vi "Perform Action on Target.vi"(8 "error in":errorcluster, 9 "Input":variant, 10 "Task-Point Ident":string, 11 "Series Actor in":refnum<class "Series Actor.lvclass">) -> (0 "error out":errorcluster, 1 "Output":variant, 3 "Series Actor out":refnum<class "Series Actor.lvclass">)   [LabVIEW 2023, in "Series Actor.lvlib" / "Series Actor.lvclass"]
uses:
  Series Actor.lvclass
  <vilib>/ActorFramework/Actor/Actor.lvclass/Actor.ctl
  Study/Study Actor/IStudy Actor Messages/Perform Action on Target Msg/Perform Action on Target Msg.lvclass/Perform Action on Target Msg.ctl
  <vilib>/ActorFramework/Reply Msg/Reply Msg.lvclass/Reply Msg.ctl
  <vilib>/ActorFramework/Message Enqueuer/Message Enqueuer.lvclass/Message Enqueuer.ctl
  <vilib>/ActorFramework/Reply Msg/Send Message And Wait For Response.vi
  <vilib>/ActorFramework/Message Enqueuer/Enqueue.vi
  Study/Study Actor/IStudy Actor Messages/Perform Action on Target Msg/Perform Action on Target Msg.lvclass
  <vilib>/ActorFramework/Reply Msg/Reply Msg.lvclass
  <vilib>/Utility/LVClass/Get LV Class Name.vi
  <resource>/AFDebug/Generate Trace for Message.vi
  <vilib>/ActorFramework/Message Priority Queue/Priority Enqueue.vi
  <vilib>/ActorFramework/Actor/Actor.lvclass
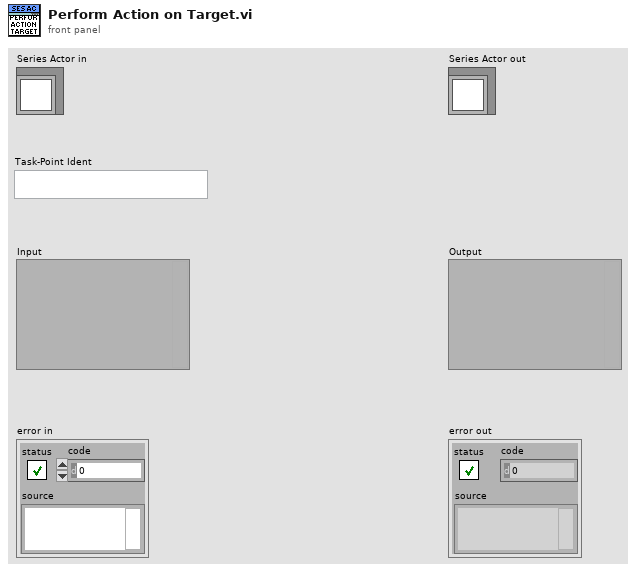
[diagram p1: front panel]
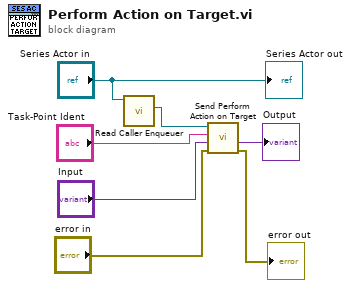
[diagram p0: block diagram]
diagram:
  n1 = call <vilib>:"Read Caller Enqueuer.vi"("Actor"="Series Actor in") -> ("Caller Enqueuer"=w4:refnum<class "Message Enqueuer.lvclass">)  [unwired: 10 in]
  n2 = call "Send Perform Action on Target.vi"("error in"="error in", "Input"="Input", "Task-Point Ident"="Task-Point Ident", "Message Enqueuer"=w4) -> ("error out"=→"error out":errorcluster, "Output"=→"Output":variant)  [unwired: 5 in, 1 out]
  "Series Actor out" <- "Series Actor in"
